vi "TF_Mech_system.vi"() -> ()   [LabVIEW 2019]
uses:
  <vilib>/addons/Control Design/_Model Construction/Model Creation.llb/Model Creation SubVI/cd_Create Transfer Function Model.vi
  <vilib>/addons/Control Design/_Time Response Analysis/Time Response.llb/Time Response subVI/cd_Impulse Response (Transfer Function).vi
  <vilib>/addons/Control Design/_Time Response Analysis/Time Response.llb/Time Response subVI/cd_Step Response (Transfer Function).vi
  <vilib>/addons/Control Design/_Utility/Model Viewer.llb/Model Viewer SubVI/cd_Draw Transfer Function Equation (TF).vi
  <vilib>/addons/Control Design/_Model Construction/NI_LinSys_Model Creation.lvlib
  <vilib>/addons/Control Design/_Utility/NI_CD_Model Viewer.lvlib
  <vilib>/addons/Control Design/_Time Response Analysis/NI_CD_Time Response.lvlib
panel:
  in  "s4":dbl(slide) scale=0.0..1.0
  in  "s3":dbl(slide) scale=0.0..1.0
  in  "s2":dbl(slide) scale=0.0..1.0
  in  "s1":dbl(slide) scale=0.0..1.0
  in  "s0":dbl(slide) scale=0.0..1.0
  in  "n1":dbl(slide) scale=0.0..1.0
  in  "n0":dbl(slide) scale=0.0..1.0
  out "Impulse Response Graph":cluster{"time":dbl[], dbl[]}[](graph)
  out "Step Response Graph":cluster{"time":dbl[], dbl[]}[](graph)
  out "Transfer Function":picture
  out "Numerator":dbl[](array[numeric])
  out "Denominator":dbl[](array[numeric])
  in  "K3":dbl(slide) scale=0.0..100.0
  in  "B":dbl(slide) scale=0.0..100.0
  in  "K2":dbl(slide) scale=0.0..100.0
  in  "K1":dbl(slide) scale=0.0..100.0
  in  "M2":dbl(slide) scale=0.0..100.0
  in  "M1":dbl(slide) scale=0.0..100.0
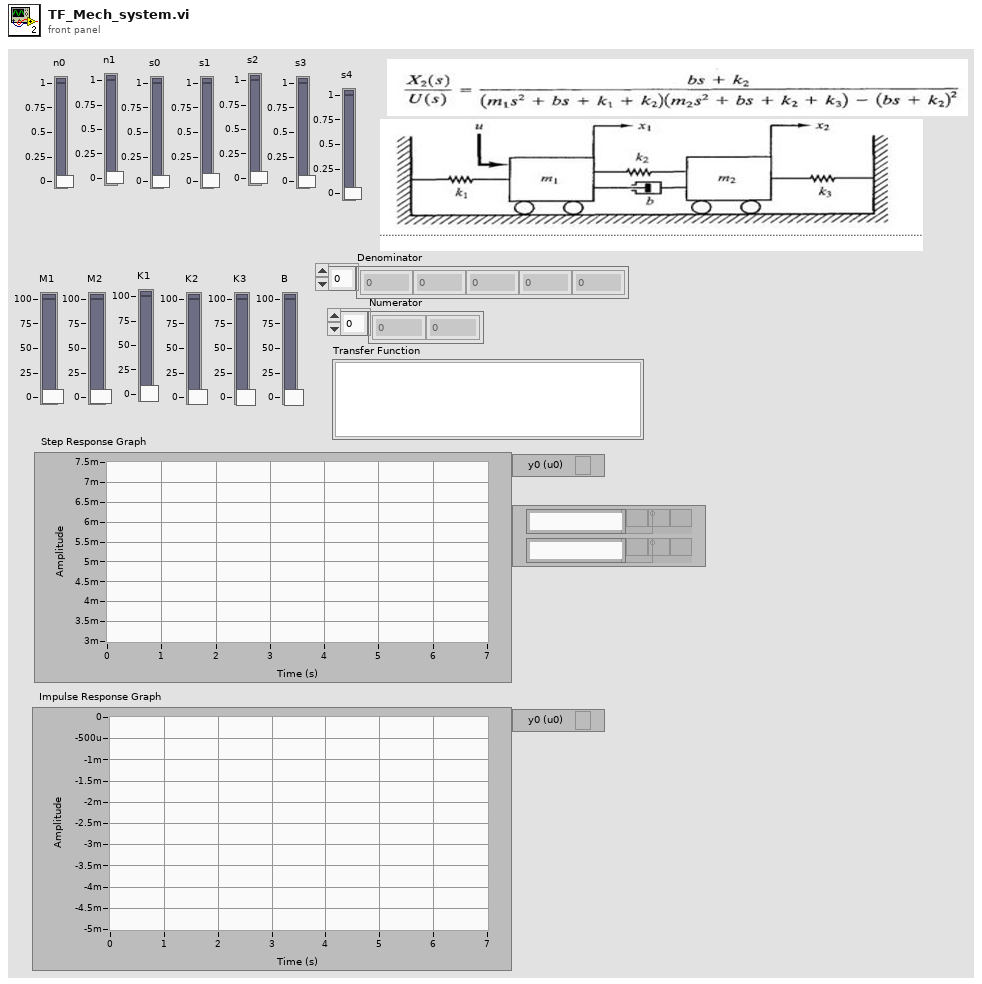
[diagram p1: front panel]
types:
  T1 = typedef "NI_LinSys_Model Typedefs.lvlib/CD Transfer Function Model (MIMO).ctl" = cluster{"properties":T2, "transfer function(s)":T3[][]}
  T2 = typedef "NI_LinSys_Model Typedefs.lvlib/CD General Elements.ctl" = cluster{"Model name":string, "Input names":string[], "Output names":string[], "Input Delays":dbl[], "Output Delays":dbl[], "Sampling Time":dbl, "Notes":string}
  T3 = typedef "NI_LinSys_Model Typedefs.lvlib/CD Transfer Function Model (SISO).ctl" = cluster{"Numerator":dbl[], "Denominator":dbl[], "delay":dbl}
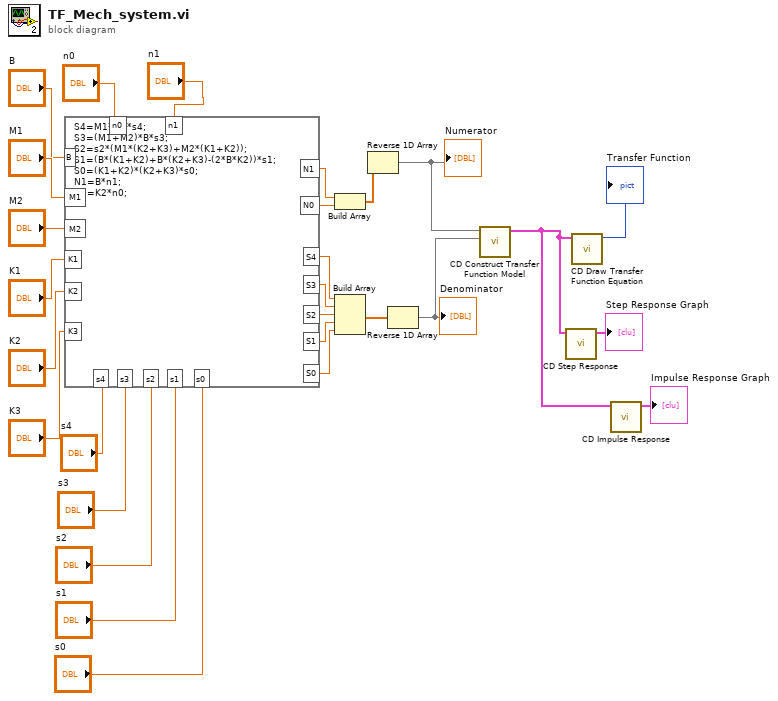
[diagram p0: block diagram]
diagram:
  n1 = formula code="S4=M1*M2*s4;\nS3=(M1+M2)*B*s3;\nS2=s2*(M1*(K2+K3)+M2*(K1+K2));\nS1=(B*(K1+K2)+B*(K2+K3)-(2*B*K2))*s1;\nS0=(K1+K2)*(K2+K3)*s0;\nN1=B*n1;\nN0=K2*n0;"("B"="B", "M1"="M1", "M2"="M2", "K1"="K1", "K2"="K2", "K3"="K3", "s4"="s4", "s3"="s3", "s2"="s2", "s1"="s1", "s0"="s0", "n0"="n0", "n1"="n1") -> ("N1"=w22:dbl, "N0"=w21:dbl, "S4"=w20:dbl, "S3"=w19:dbl, "S2"=w18:dbl, "S1"=w17:dbl, "S0"=w16:dbl)
  n2 = Build Array(w22, w21) -> (w14:dbl[])
  n3 = Build Array(w20, w19, w18, w17, w16) -> (w13:dbl[])
  n4 = Reverse 1D Array(array=w14) -> (reversed array=w8:dbl[])
  "Numerator" <- w8
  n5 = Reverse 1D Array(array=w13) -> (reversed array=w12:dbl[])
  "Denominator" <- w12
  n6 = call-poly <vilib>:"CD Construct Transfer Function Model.vi"("Denominator"=w12, "Numerator"=w8) -> ("Transfer Function Model"=w9:T1)  [unwired: 8 in, 1 out]
  n7 = call-poly <vilib>:"CD Step Response.vi"("Transfer Function Model"=w9) -> ("Step Response Graph"=→"Step Response Graph":cluster{"time":dbl[], dbl[]}[])  [unwired: 8 in, 2 out]
  n8 = call-poly <vilib>:"CD Draw Transfer Function Equation.vi"("Transfer Function Model"=w9) -> ("Equation"=→"Transfer Function":picture)  [unwired: 8 in, 2 out]
  n9 = call-poly <vilib>:"CD Impulse Response.vi"("Transfer Function Model"=w9) -> ("Impulse Response Graph"=→"Impulse Response Graph":cluster{"time":dbl[], dbl[]}[])  [unwired: 8 in, 2 out]
